vi "RefreshAutoUI.vi"(0 "TestDataRefs":refnum<vi>[](array[refnum]), 1 "RefreshAutoUIFunc":T3, 5 "CtrlPanelRefs":refnum<vi>[](array[refnum]), 7 "PIDCtrlRefs":refnum<vi>[](array[refnum]), 9 "OtherCtrlRefs":refnum<vi>[](array[refnum]), 11 "RecipeCtrlRefs":refnum<vi>[](array[refnum]), 12 "Setting":T1={"TorqueSensor"={"Interface"="", "Read Unit"=enum."Kg.cm", "Encoder"=0, "Torque Filter"=0, "Max Torque"=2.0, "Max Power"=50.0, "Max Speed"=50.0, "Scale Factor CW"=2.0, "Scale Factor CCW"=2.0, "Scale Factor Zero"=2.0}, "TorqueSensorL"={"Interface"="", "Read Unit"=enum."Kg.cm", "Encoder"=0, "Torque Filter"=0, "Max Torque"=2.0, "Max Power"=50.0, "Max Speed"=50.0, "Scale Factor CW"=2.0, "Scale Factor CCW"=2.0, "Scale Factor Zero"=2.0}, "Power Meter"={"Wiring"=0, "Interface"="", "1P Mode"=1, "1P CurrentLimit"=0.0, "3P Mode"=1, "3P CurrentLimit"=0.0}, "Thermocouple"={"Interface"="", "value range"="T/C T type -100 ~ 400 degree C", "Channel Count"=8, "Limit 0"=0.0, "Limit 1"=0.0, "Limit 2"=0.0, "Limit 3"=0.0, "Limit 4"=0.0, "Limit 5"=0.0, "Limit 6"=0.0, "Limit 7"=0.0}, "DC-1000"={"Interface"=enum."AD-1"}, "ServoMotor"={"Interface"=enum."AD-1"}, "MotorDriver"={"D_Interface"="", "L_Interface"=""}, "TestMode"=enum."電子中軸測試", "PowerSupply"={"Interface"="", "Current"=50.0, "Voltage"=50.0}} {"Thermocouple"."Limit 7" format="%.1f"; "Thermocouple"."Limit 6" format="%.1f"; "Thermocouple"."Limit 5" format="%.1f"; "Thermocouple"."Limit 4" format="%.1f"; "Thermocouple"."Limit 3" format="%.1f"; "Thermocouple"."Limit 2" format="%.1f"; "Thermocouple"."Limit 1" format="%.1f"; "Thermocouple"."Limit 0" format="%.1f"; "Thermocouple"."Channel Count" min=0 max=24; "Power Meter"."3P Mode" items=["RMS", "MEAN", "DC"]; "Power Meter"."1P Mode" items=["RMS", "MEAN", "DC"]; "Power Meter"."Wiring" items=["AD-0", "AD-1"]; "TorqueSensorL"."Scale Factor Zero" format="%#.6f"; "TorqueSensorL"."Scale Factor CCW" format="%#.6f"; "TorqueSensorL"."Scale Factor CW" format="%#.6f"; "TorqueSensorL"."Torque Filter" items=["OFF", "10Hz", "25Hz", "50Hz", "3Hz", "2Hz", "1Hz"]; "TorqueSensorL"."Encoder" items=["60-ppr"=60, "600-ppr"=600, "6000-ppr"=6000, "8192-ppr"=8192, "20-ppr"=20, "30-ppr"=30, "1-ppr"=1, "2-ppr"=2, "6-ppr"=6]; "TorqueSensor"."Scale Factor Zero" format="%#.6f"; "TorqueSensor"."Scale Factor CCW" format="%#.6f"; "TorqueSensor"."Scale Factor CW" format="%#.6f"; "TorqueSensor"."Torque Filter" items=["OFF", "10Hz", "25Hz", "50Hz", "3Hz", "2Hz", "1Hz"]; "TorqueSensor"."Encoder" items=["60-ppr"=60, "600-ppr"=600, "6000-ppr"=6000, "8192-ppr"=8192, "20-ppr"=20, "30-ppr"=30, "1-ppr"=1, "2-ppr"=2, "6-ppr"=6]}) -> ()   [LabVIEW 2024]
uses:
  RefreshAutoUIFunc.ctl
  MFActor/SystemSettings.ctl
panel:
  in  "Tab Control":T2(tab)
  in  "TestDataCurve":refnum<vi>
  in  "YAxis":refnum<vi>
  in  "XAxis":refnum<vi>
  in  "tbTestData":refnum<vi>
  in  "PIDGraph":refnum<vi>
  in  "pgTestData":refnum<vi>
  in  "ZeroLoadTorque":refnum<vi>
  in  "ZeroDriveTorque":refnum<vi>
  in  "ZeroDriveSpeed":refnum<vi>
  in  "LoadServoOn":refnum<vi>
  in  "DriveServoOn":refnum<vi>
  in  "TQOutput_L":refnum<vi>
  in  "SpeedOutput_D":refnum<vi>
  in  "CWCCW":refnum<vi>
  in  "pgCtrlPanel":refnum<vi>
  in  "TQOutput_D":refnum<vi>
  in  "OkeyForPID":refnum<vi>
  in  "PID Adj.End":refnum<vi>
  in  "PID Adj.Start":refnum<vi>
  in  "Close Loop Value Lo":refnum<vi>
  in  "Close Loop Value Hi":refnum<vi>
  in  "Close Loop Value Dwell":refnum<vi>
  in  "Close Loop Value Speed":refnum<vi>
  in  "NDS":refnum<vi>
  in  "NIS":refnum<vi>
  in  "NPS":refnum<vi>
  in  "ND":refnum<vi>
  in  "NI":refnum<vi>
  in  "NP":refnum<vi>
  in  "StopTest":refnum<vi>
  in  "StartTest":refnum<vi>
  in  "GotoCurvePage":refnum<vi>
  in  "GotoDataPage":refnum<vi>
  in  "ZeroDegree":refnum<vi>
  in  "ProcessConfirm":refnum<vi>
  in  "DynoValue_Auto":refnum<vi>
  in  "TestPanel":refnum<vi>
  in  "Trugh":refnum<vi>
  in  "LoadSideTQ":refnum<vi>
  in  "SinWaveTestSpeed":refnum<vi>
  in  "DegSetValue":refnum<vi>
  in  "TorqueSettingValue":refnum<vi>
  in  "Crest":refnum<vi>
  in  "PIDAdj":refnum<vi>
  in  "PID":refnum<vi>
  in  "MultiPtInitSpeed":refnum<vi>
  in  "Remove Button":refnum<vi>
  in  "Insert Button":refnum<vi>
  in  "Modify Button":refnum<vi>
  in  "Add Button":refnum<vi>
  in  "mtpTorque":refnum<vi>
  in  "mtpFetchRate":refnum<vi>
  in  "mtpDwellTime":refnum<vi>
  in  "mtpSpeed":refnum<vi>
  in  "idx":refnum<vi>
  in  "Program_Multi":refnum<vi>
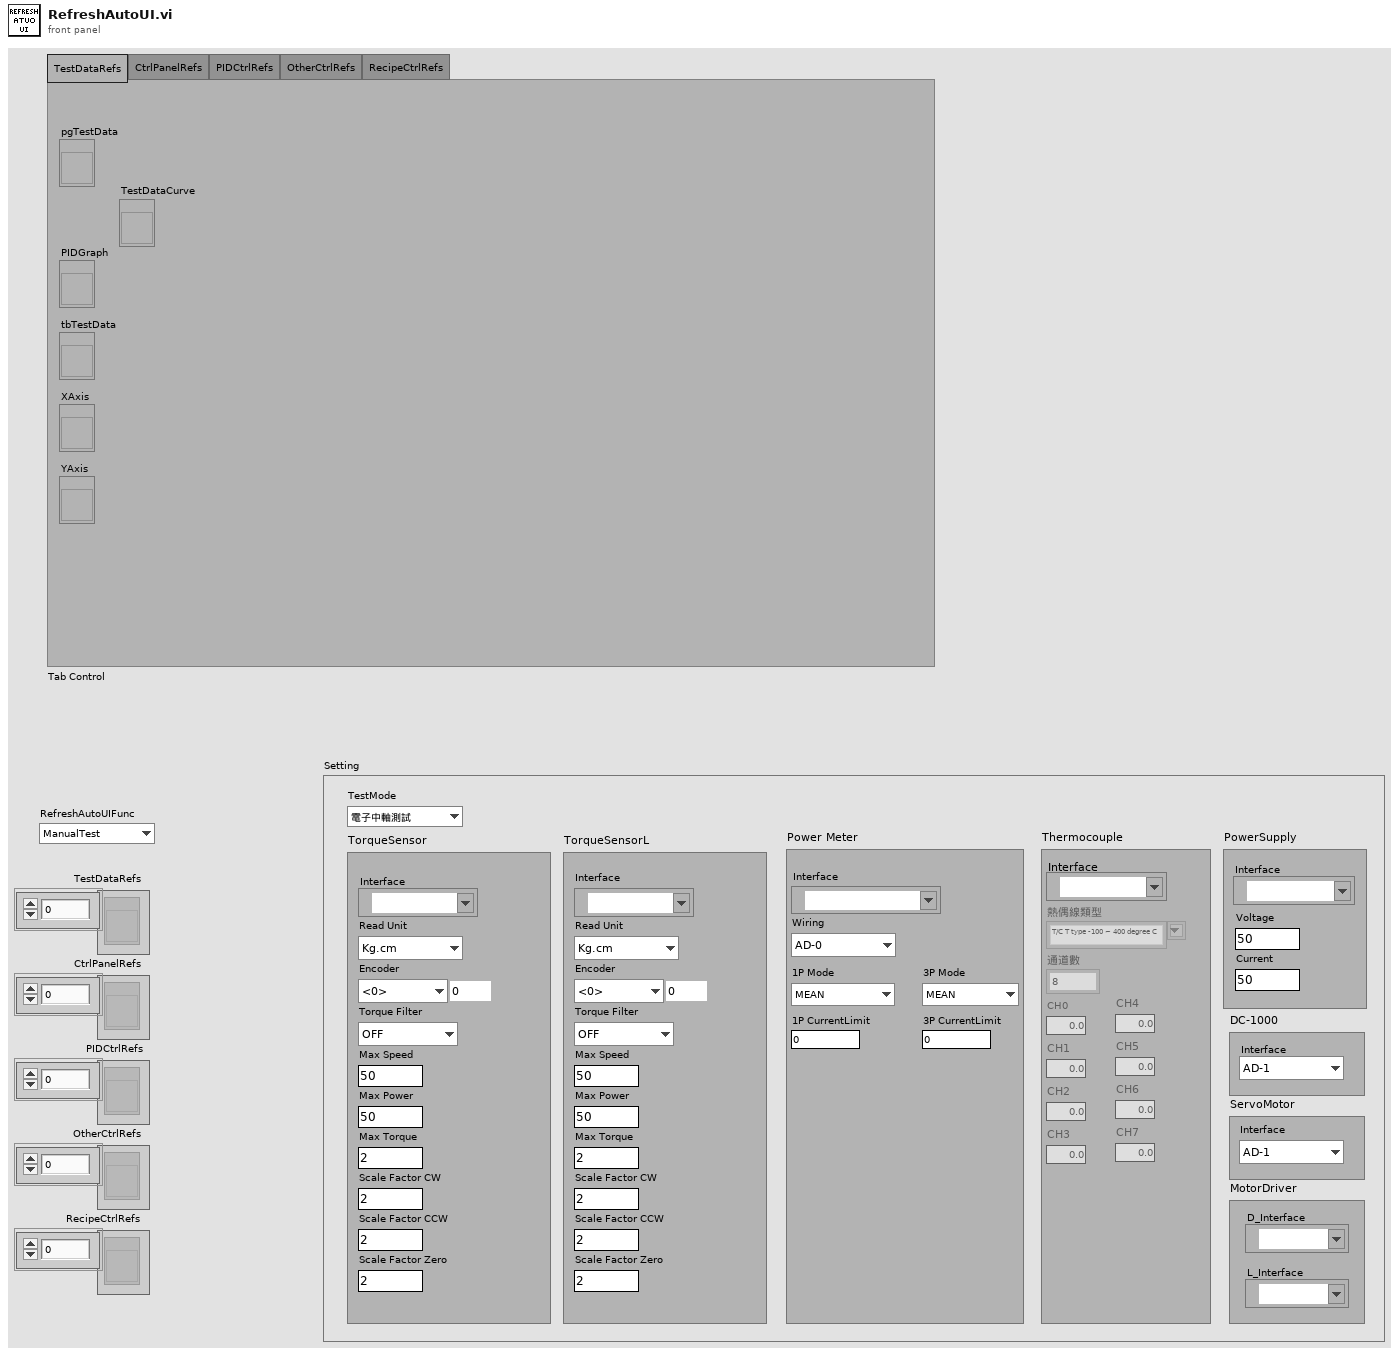
[diagram p1: front panel]
types:
  T1 = typedef "SystemSettings.ctl" = cluster{"TorqueSensor":cluster{"Interface":refnum<visa-resource-name>, "Read Unit":enum16{"oz.in", "oz.ft", "lb.in", "lb.ft", "g.cm", "Kg.cm", "mN.m", "cN.m", "N.m"}, "Encoder":u16, "Torque Filter":u16, "Max Torque":dbl, "Max Power":dbl, "Max Speed":dbl, "Scale Factor CW":dbl, "Scale Factor CCW":dbl, "Scale Factor Zero":dbl}, "TorqueSensorL":cluster{"Interface":refnum<visa-resource-name>, "Read Unit":enum16{"oz.in", "oz.ft", "lb.in", "lb.ft", "g.cm", "Kg.cm", "mN.m", "cN.m", "N.m"}, "Encoder":u16, "Torque Filter":u16, "Max Torque":dbl, "Max Power":dbl, "Max Speed":dbl, "Scale Factor CW":dbl, "Scale Factor CCW":dbl, "Scale Factor Zero":dbl}, "Power Meter":cluster{"Wiring":u16, "Interface":refnum<visa-resource-name>, "1P Mode":u16, "1P CurrentLimit":dbl, "3P Mode":u16, "3P CurrentLimit":dbl}, "Thermocouple":cluster{"Interface":refnum<visa-resource-name>, "value range":string, "Channel Count":i32, "Limit 0":dbl, "Limit 1":dbl, "Limit 2":dbl, "Limit 3":dbl, "Limit 4":dbl, "Limit 5":dbl, "Limit 6":dbl, "Limit 7":dbl}, "DC-1000":cluster{"Interface":enum16{"AD-0", "AD-1"}}, "ServoMotor":cluster{"Interface":enum16{"AD-0", "AD-1"}}, "MotorDriver":cluster{"D_Interface":refnum<visa-resource-name>, "L_Interface":refnum<visa-resource-name>}, "TestMode":enum16{"電子中軸測試", "中置電機測試"}, "PowerSupply":cluster{"Interface":refnum<visa-resource-name>, "Current":dbl, "Voltage":dbl}}
  T2 = enum32{"TestDataRefs", "CtrlPanelRefs", "PIDCtrlRefs", "OtherCtrlRefs", "RecipeCtrlRefs"}
  T3 = typedef "RefreshAutoUIFunc.ctl" = enum16{"ManualTest", "AngleMode", "LoadWaveCtrlMode", "DriveWaveCtrlMode", "EditMultiPt", "MultiPtTestMode", "FixPtTestMode", "AdjPID", "ConfirmBtnPos"}
  T4 = enum8{"Enabled", "Disabled", "Disabled and Grayed Out"}
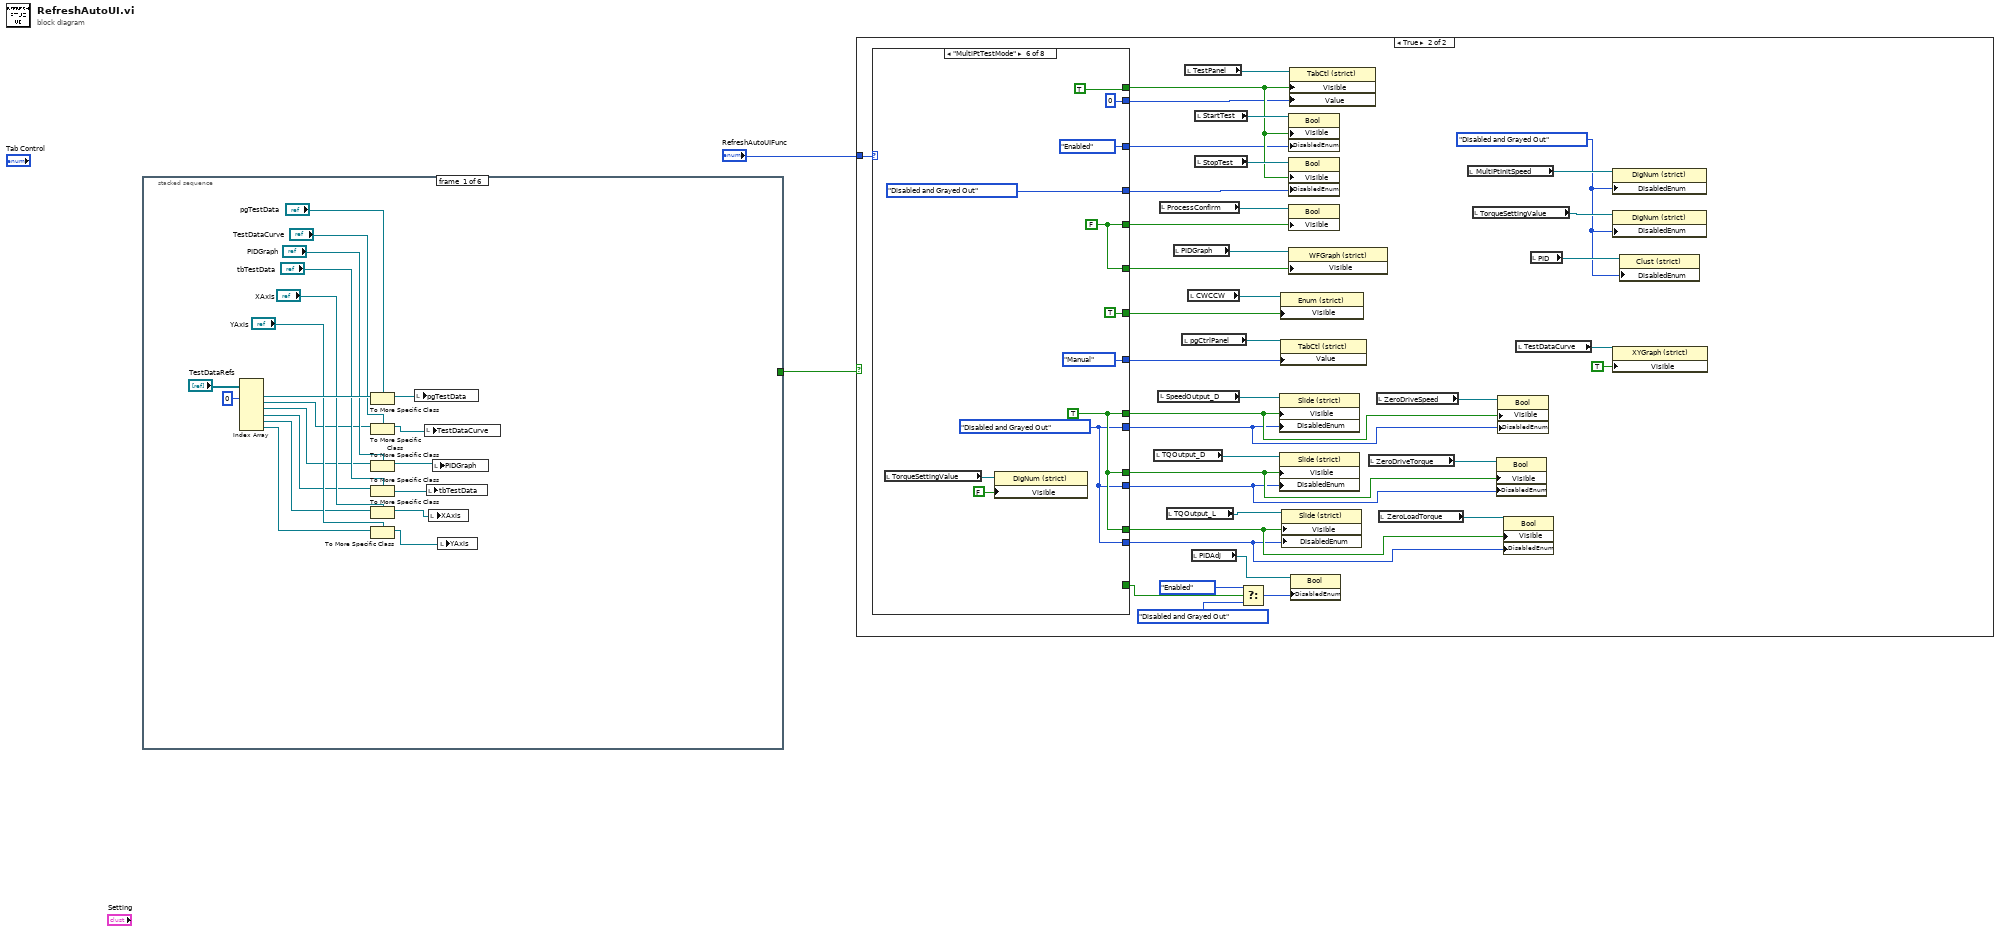
[diagram p0: block diagram]
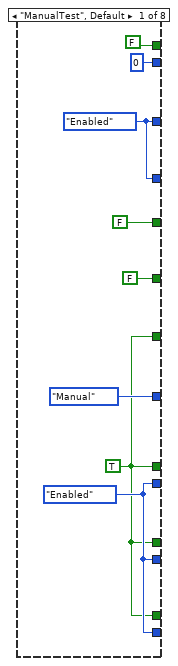
[diagram p3: hidden frame]
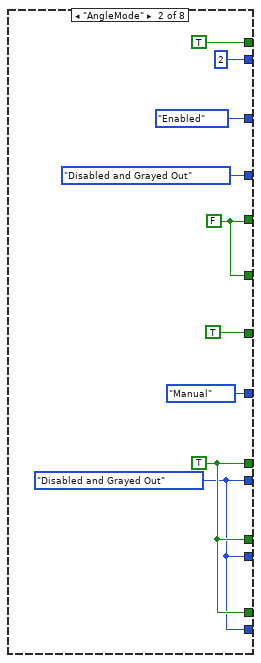
[diagram p4: hidden frame]
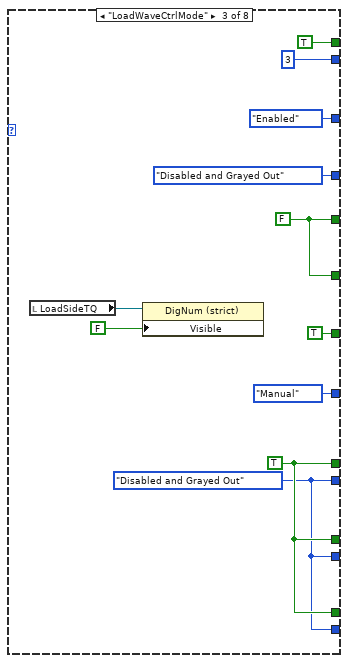
[diagram p5: hidden frame]
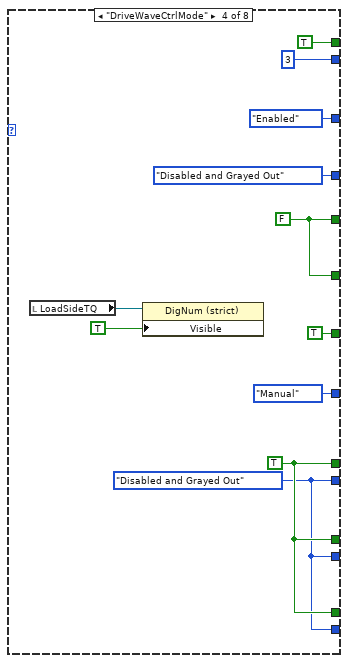
[diagram p6: hidden frame]
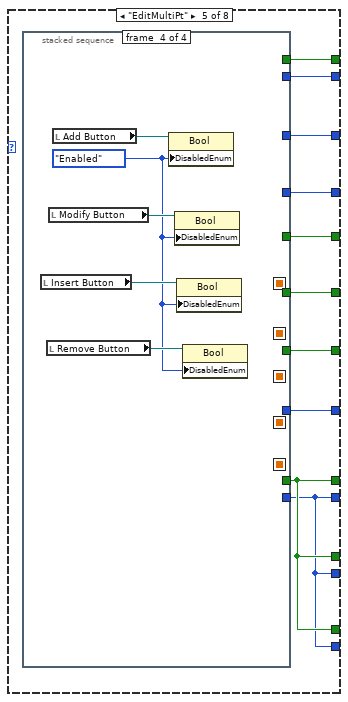
[diagram p7: hidden frame]
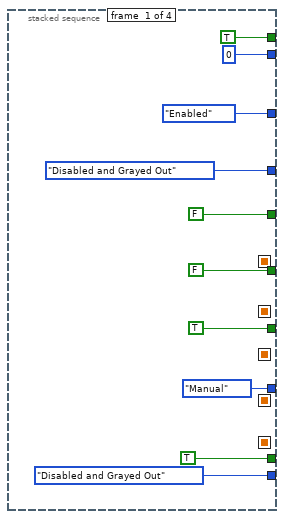
[diagram p8: hidden frame]
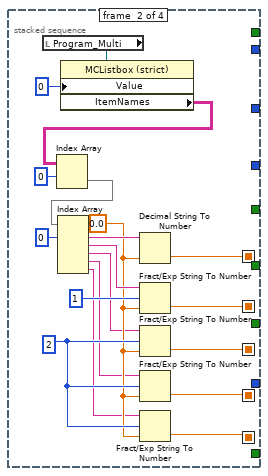
[diagram p9: hidden frame]
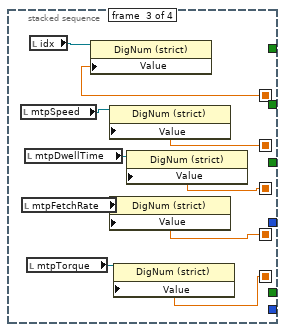
[diagram p10: hidden frame]
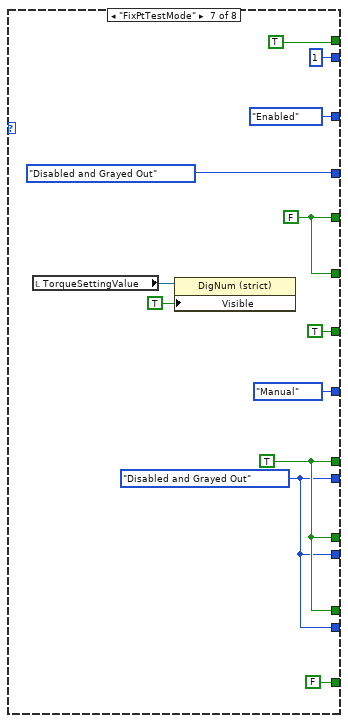
[diagram p11: hidden frame]
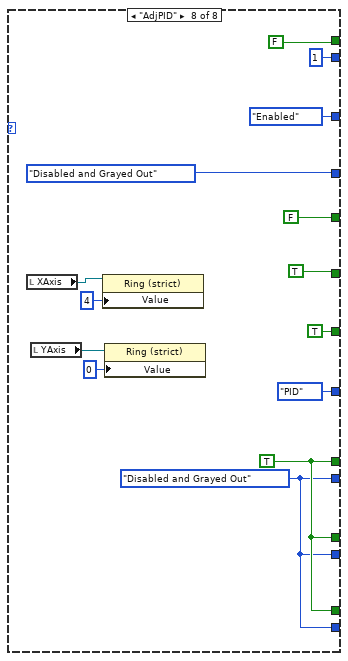
[diagram p12: hidden frame]
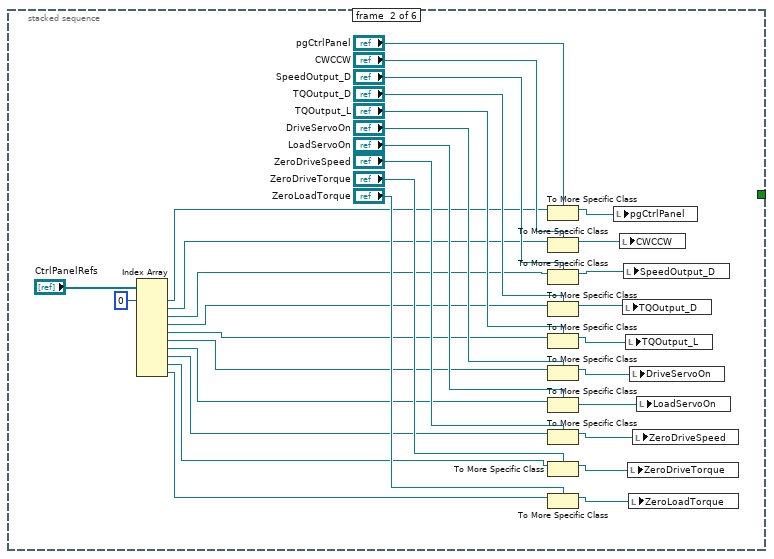
[diagram p13: hidden frame]
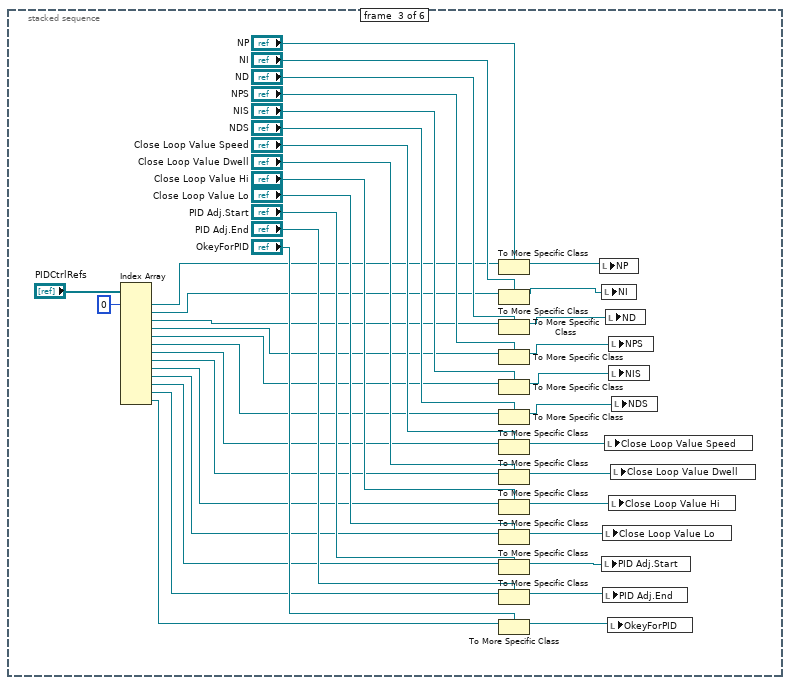
[diagram p14: hidden frame]
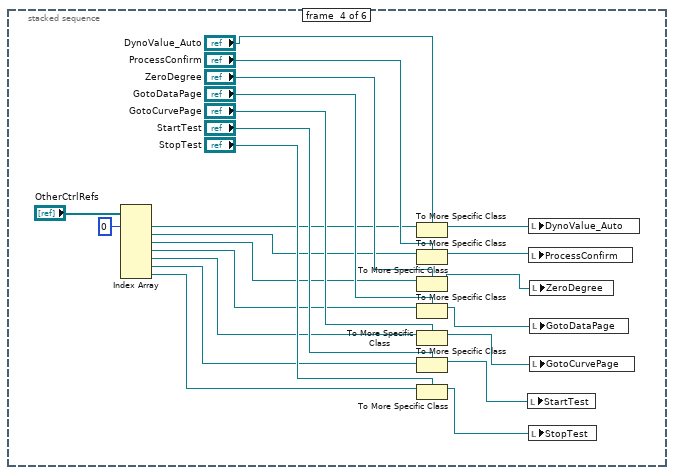
[diagram p15: hidden frame]
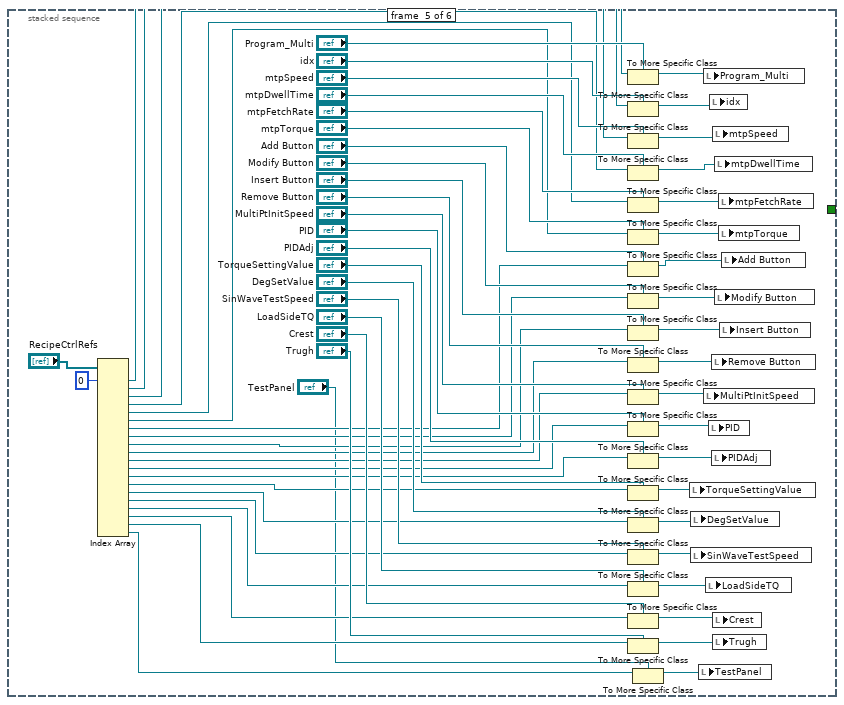
[diagram p16: hidden frame]
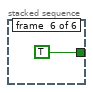
[diagram p17: hidden frame]
diagram:
  n1 = stacked-sequence {
    tunnel: [_ _ _ _ _ TRUE] -> w2
    frame #0 {
      n2 = Index Array(array="TestDataRefs", index #1=0 ("index")) -> (element #1=w20:refnum<vi>, element #2=w3:refnum<vi>, element #3=w4:refnum<vi>, element #4=w5:refnum<vi>, element #5=w6:refnum<vi>, element #6=w7:refnum<vi>)  [unwired: 5 in]
      n3 = To More Specific Class(target class="pgTestData", reference=w20) -> (specific class reference=w19:refnum<vi>)  [unwired: 1 in, 1 out]
      n4 = To More Specific Class(target class="TestDataCurve", reference=w3) -> (specific class reference=w9:refnum<vi>)  [unwired: 1 in, 1 out]
      n5 = To More Specific Class(target class="PIDGraph", reference=w4) -> (specific class reference=w15:refnum<vi>)  [unwired: 1 in, 1 out]
      n6 = To More Specific Class(target class="tbTestData", reference=w5) -> (specific class reference=w14:refnum<vi>)  [unwired: 1 in, 1 out]
      n7 = To More Specific Class(target class="XAxis", reference=w6) -> (specific class reference=w13:refnum<vi>)  [unwired: 1 in, 1 out]
      n8 = To More Specific Class(target class="YAxis", reference=w7) -> (specific class reference=w12:refnum<vi>)  [unwired: 1 in, 1 out]
      n9 = local write "pgTestData"(w19) -> ()
      n10 = local write "TestDataCurve"(w9) -> ()
      n11 = local write "tbTestData"(w14) -> ()
      n12 = local write "XAxis"(w13) -> ()
      n13 = local write "PIDGraph"(w15) -> ()
      n14 = local write "YAxis"(w12) -> ()
    }
    frame #1 {
      n15 = Index Array(array="CtrlPanelRefs", index #1=0 ("index")) -> (element #1=w32:refnum<vi>, element #2=w31:refnum<vi>, element #3=w30:refnum<vi>, element #4=w29:refnum<vi>, element #5=w28:refnum<vi>, element #6=w27:refnum<vi>, element #7=w26:refnum<vi>, element #8=w25:refnum<vi>, element #9=w24:refnum<vi>, element #10=w23:refnum<vi>)  [unwired: 9 in]
      n16 = To More Specific Class(target class="pgCtrlPanel", reference=w32) -> (specific class reference=w42:refnum<vi>)  [unwired: 1 in, 1 out]
      n17 = To More Specific Class(target class="CWCCW", reference=w31) -> (specific class reference=w41:refnum<vi>)  [unwired: 1 in, 1 out]
      n18 = To More Specific Class(target class="SpeedOutput_D", reference=w30) -> (specific class reference=w40:refnum<vi>)  [unwired: 1 in, 1 out]
      n19 = To More Specific Class(target class="TQOutput_D", reference=w29) -> (specific class reference=w39:refnum<vi>)  [unwired: 1 in, 1 out]
      n20 = To More Specific Class(target class="TQOutput_L", reference=w28) -> (specific class reference=w38:refnum<vi>)  [unwired: 1 in, 1 out]
      n21 = To More Specific Class(target class="DriveServoOn", reference=w27) -> (specific class reference=w37:refnum<vi>)  [unwired: 1 in, 1 out]
      n22 = To More Specific Class(target class="LoadServoOn", reference=w26) -> (specific class reference=w36:refnum<vi>)  [unwired: 1 in, 1 out]
      n23 = To More Specific Class(target class="ZeroDriveSpeed", reference=w25) -> (specific class reference=w35:refnum<vi>)  [unwired: 1 in, 1 out]
      n24 = To More Specific Class(target class="ZeroDriveTorque", reference=w24) -> (specific class reference=w34:refnum<vi>)  [unwired: 1 in, 1 out]
      n25 = To More Specific Class(target class="ZeroLoadTorque", reference=w23) -> (specific class reference=w33:refnum<vi>)  [unwired: 1 in, 1 out]
      n26 = local write "pgCtrlPanel"(w42) -> ()
      n27 = local write "CWCCW"(w41) -> ()
      n28 = local write "TQOutput_D"(w39) -> ()
      n29 = local write "SpeedOutput_D"(w40) -> ()
      n30 = local write "TQOutput_L"(w38) -> ()
      n31 = local write "ZeroDriveTorque"(w34) -> ()
      n32 = local write "ZeroLoadTorque"(w33) -> ()
      n33 = local write "DriveServoOn"(w37) -> ()
      n34 = local write "ZeroDriveSpeed"(w35) -> ()
      n35 = local write "LoadServoOn"(w36) -> ()
    }
    frame #2 {
      n36 = Index Array(array="PIDCtrlRefs", index #1=0 ("index")) -> (element #1=w80:refnum<vi>, element #2=w79:refnum<vi>, element #3=w78:refnum<vi>, element #4=w77:refnum<vi>, element #5=w76:refnum<vi>, element #6=w75:refnum<vi>, element #7=w74:refnum<vi>, element #8=w73:refnum<vi>, element #9=w72:refnum<vi>, element #10=w71:refnum<vi>, element #11=w70:refnum<vi>, element #12=w69:refnum<vi>, element #13=w68:refnum<vi>)  [unwired: 12 in]
      n37 = To More Specific Class(target class="NP", reference=w80) -> (specific class reference=w67:refnum<vi>)  [unwired: 1 in, 1 out]
      n38 = To More Specific Class(target class="NI", reference=w79) -> (specific class reference=w66:refnum<vi>)  [unwired: 1 in, 1 out]
      n39 = To More Specific Class(target class="ND", reference=w78) -> (specific class reference=w65:refnum<vi>)  [unwired: 1 in, 1 out]
      n40 = To More Specific Class(target class="NPS", reference=w77) -> (specific class reference=w64:refnum<vi>)  [unwired: 1 in, 1 out]
      n41 = To More Specific Class(target class="NIS", reference=w76) -> (specific class reference=w63:refnum<vi>)  [unwired: 1 in, 1 out]
      n42 = To More Specific Class(target class="NDS", reference=w75) -> (specific class reference=w62:refnum<vi>)  [unwired: 1 in, 1 out]
      n43 = To More Specific Class(target class="Close Loop Value Speed", reference=w74) -> (specific class reference=w61:refnum<vi>)  [unwired: 1 in, 1 out]
      n44 = To More Specific Class(target class="Close Loop Value Dwell", reference=w73) -> (specific class reference=w60:refnum<vi>)  [unwired: 1 in, 1 out]
      n45 = To More Specific Class(target class="Close Loop Value Hi", reference=w72) -> (specific class reference=w59:refnum<vi>)  [unwired: 1 in, 1 out]
      n46 = To More Specific Class(target class="Close Loop Value Lo", reference=w71) -> (specific class reference=w58:refnum<vi>)  [unwired: 1 in, 1 out]
      n47 = To More Specific Class(target class="PID Adj.Start", reference=w70) -> (specific class reference=w57:refnum<vi>)  [unwired: 1 in, 1 out]
      n48 = To More Specific Class(target class="PID Adj.End", reference=w69) -> (specific class reference=w56:refnum<vi>)  [unwired: 1 in, 1 out]
      n49 = To More Specific Class(target class="OkeyForPID", reference=w68) -> (specific class reference=w55:refnum<vi>)  [unwired: 1 in, 1 out]
      n50 = local write "NP"(w67) -> ()
      n51 = local write "NI"(w66) -> ()
      n52 = local write "PID Adj.Start"(w57) -> ()
      n53 = local write "Close Loop Value Lo"(w58) -> ()
      n54 = local write "PID Adj.End"(w56) -> ()
      n55 = local write "Close Loop Value Speed"(w61) -> ()
      n56 = local write "ND"(w65) -> ()
      n57 = local write "OkeyForPID"(w55) -> ()
      n58 = local write "NPS"(w64) -> ()
      n59 = local write "NIS"(w63) -> ()
      n60 = local write "Close Loop Value Hi"(w59) -> ()
      n61 = local write "Close Loop Value Dwell"(w60) -> ()
      n62 = local write "NDS"(w62) -> ()
    }
    frame #3 {
      n63 = Index Array(array="OtherCtrlRefs", index #1=0 ("index")) -> (element #1=w109:refnum<vi>, element #2=w108:refnum<vi>, element #3=w107:refnum<vi>, element #4=w106:refnum<vi>, element #5=w105:refnum<vi>, element #6=w104:refnum<vi>, element #7=w103:refnum<vi>)  [unwired: 6 in]
      n64 = To More Specific Class(target class="DynoValue_Auto", reference=w109) -> (specific class reference=w102:refnum<vi>)  [unwired: 1 in, 1 out]
      n65 = To More Specific Class(target class="ProcessConfirm", reference=w108) -> (specific class reference=w101:refnum<vi>)  [unwired: 1 in, 1 out]
      n66 = To More Specific Class(target class="ZeroDegree", reference=w107) -> (specific class reference=w100:refnum<vi>)  [unwired: 1 in, 1 out]
      n67 = To More Specific Class(target class="GotoDataPage", reference=w106) -> (specific class reference=w99:refnum<vi>)  [unwired: 1 in, 1 out]
      n68 = To More Specific Class(target class="GotoCurvePage", reference=w105) -> (specific class reference=w98:refnum<vi>)  [unwired: 1 in, 1 out]
      n69 = To More Specific Class(target class="StartTest", reference=w104) -> (specific class reference=w97:refnum<vi>)  [unwired: 1 in, 1 out]
      n70 = To More Specific Class(target class="StopTest", reference=w103) -> (specific class reference=w96:refnum<vi>)  [unwired: 1 in, 1 out]
      n71 = local write "StartTest"(w97) -> ()
      n72 = local write "DynoValue_Auto"(w102) -> ()
      n73 = local write "ProcessConfirm"(w101) -> ()
      n74 = local write "StopTest"(w96) -> ()
      n75 = local write "ZeroDegree"(w100) -> ()
      n76 = local write "GotoDataPage"(w99) -> ()
      n77 = local write "GotoCurvePage"(w98) -> ()
    }
    frame #4 {
      n78 = Index Array(array="RecipeCtrlRefs", index #1=0 ("index")) -> (element #1=w159:refnum<vi>, element #2=w158:refnum<vi>, element #3=w157:refnum<vi>, element #4=w156:refnum<vi>, element #5=w155:refnum<vi>, element #6=w154:refnum<vi>, element #7=w153:refnum<vi>, element #8=w152:refnum<vi>, element #9=w151:refnum<vi>, element #10=w150:refnum<vi>, element #11=w149:refnum<vi>, element #12=w148:refnum<vi>, element #13=w147:refnum<vi>, element #14=w146:refnum<vi>, element #15=w145:refnum<vi>, element #16=w144:refnum<vi>, element #17=w143:refnum<vi>, element #18=w142:refnum<vi>, element #19=w141:refnum<vi>, element #20=w120:refnum<vi>)  [unwired: 19 in]
      n79 = To More Specific Class(target class="Program_Multi", reference=w159) -> (specific class reference=w140:refnum<vi>)  [unwired: 1 in, 1 out]
      n80 = To More Specific Class(target class="idx", reference=w158) -> (specific class reference=w139:refnum<vi>)  [unwired: 1 in, 1 out]
      n81 = To More Specific Class(target class="mtpSpeed", reference=w157) -> (specific class reference=w138:refnum<vi>)  [unwired: 1 in, 1 out]
      n82 = To More Specific Class(target class="mtpDwellTime", reference=w156) -> (specific class reference=w137:refnum<vi>)  [unwired: 1 in, 1 out]
      n83 = To More Specific Class(target class="mtpFetchRate", reference=w155) -> (specific class reference=w136:refnum<vi>)  [unwired: 1 in, 1 out]
      n84 = To More Specific Class(target class="mtpTorque", reference=w154) -> (specific class reference=w135:refnum<vi>)  [unwired: 1 in, 1 out]
      n85 = To More Specific Class(target class="Add Button", reference=w153) -> (specific class reference=w134:refnum<vi>)  [unwired: 1 in, 1 out]
      n86 = To More Specific Class(target class="Modify Button", reference=w152) -> (specific class reference=w133:refnum<vi>)  [unwired: 1 in, 1 out]
      n87 = To More Specific Class(target class="Insert Button", reference=w151) -> (specific class reference=w132:refnum<vi>)  [unwired: 1 in, 1 out]
      n88 = To More Specific Class(target class="Remove Button", reference=w150) -> (specific class reference=w131:refnum<vi>)  [unwired: 1 in, 1 out]
      n89 = To More Specific Class(target class="MultiPtInitSpeed", reference=w149) -> (specific class reference=w130:refnum<vi>)  [unwired: 1 in, 1 out]
      n90 = To More Specific Class(target class="PID", reference=w148) -> (specific class reference=w129:refnum<vi>)  [unwired: 1 in, 1 out]
      n91 = To More Specific Class(target class="PIDAdj", reference=w147) -> (specific class reference=w128:refnum<vi>)  [unwired: 1 in, 1 out]
      n92 = To More Specific Class(target class="TorqueSettingValue", reference=w146) -> (specific class reference=w127:refnum<vi>)  [unwired: 1 in, 1 out]
      n93 = To More Specific Class(target class="DegSetValue", reference=w145) -> (specific class reference=w126:refnum<vi>)  [unwired: 1 in, 1 out]
      n94 = To More Specific Class(target class="SinWaveTestSpeed", reference=w144) -> (specific class reference=w125:refnum<vi>)  [unwired: 1 in, 1 out]
      n95 = To More Specific Class(target class="LoadSideTQ", reference=w143) -> (specific class reference=w124:refnum<vi>)  [unwired: 1 in, 1 out]
      n96 = To More Specific Class(target class="Crest", reference=w142) -> (specific class reference=w123:refnum<vi>)  [unwired: 1 in, 1 out]
      n97 = To More Specific Class(target class="Trugh", reference=w141) -> (specific class reference=w122:refnum<vi>)  [unwired: 1 in, 1 out]
      n98 = To More Specific Class(target class="TestPanel", reference=w120) -> (specific class reference=w119:refnum<vi>)  [unwired: 1 in, 1 out]
      n99 = local write "TorqueSettingValue"(w127) -> ()
      n100 = local write "DegSetValue"(w126) -> ()
      n101 = local write "SinWaveTestSpeed"(w125) -> ()
      n102 = local write "TestPanel"(w119) -> ()
      n103 = local write "Program_Multi"(w140) -> ()
      n104 = local write "MultiPtInitSpeed"(w130) -> ()
      n105 = local write "LoadSideTQ"(w124) -> ()
      n106 = local write "PID"(w129) -> ()
      n107 = local write "idx"(w139) -> ()
      n108 = local write "Remove Button"(w131) -> ()
      n109 = local write "PIDAdj"(w128) -> ()
      n110 = local write "mtpSpeed"(w138) -> ()
      n111 = local write "Crest"(w123) -> ()
      n112 = local write "Trugh"(w122) -> ()
      n113 = local write "mtpDwellTime"(w137) -> ()
      n114 = local write "Modify Button"(w133) -> ()
      n115 = local write "mtpFetchRate"(w136) -> ()
      n116 = local write "mtpTorque"(w135) -> ()
      n117 = local write "Insert Button"(w132) -> ()
      n118 = local write "Add Button"(w134) -> ()
    }
    frame #5 {
    }
  }
  n119 = case shown="True" w2 {
    tunnel: "RefreshAutoUIFunc" -> [_ w220]
    frame False {
    }
    frame True {
      w184 = T4."Disabled and Grayed Out" ("Disabled")
      n120 = case shown="\"MultiPtTestMode\"" w220 {
        tunnel: [FALSE TRUE TRUE TRUE w269 TRUE TRUE FALSE] -> w215
        tunnel: [FALSE w233 w244 w255 w265 w321 w333 TRUE] -> w213
        tunnel: [enum32{"Manual", "PID"}."Manual" ("Value") enum32{"Manual", "PID"}."Manual" ("Value") enum32{"Manual", "PID"}."Manual" ("Value") enum32{"Manual", "PID"}."Manual" ("Value") w263 enum32{"Manual", "PID"}."Manual" ("Value") enum32{"Manual", "PID"}."Manual" ("Value") enum32{"Manual", "PID"}."PID" ("Value")] -> w211
        tunnel: [w224 w231 w241 w252 w262 w318 w330 w344] -> w204
        tunnel: [w224 w231 w241 w252 w262 w318 w330 w344] -> w202
        tunnel: [w224 w231 w241 w252 w262 w318 w330 w344] -> w200
        tunnel: [w225 w230 w240 w251 w261 w317 w329 w343] -> w203
        tunnel: [w225 w230 w240 w251 w261 w317 w329 w343] -> w201
        tunnel: [w225 w230 w240 w251 w261 w317 w329 w343] -> w199
        tunnel: [w224 TRUE TRUE TRUE w264 TRUE TRUE TRUE] -> w197
        tunnel: [FALSE w233 w244 w255 w266 w321 w333 FALSE] -> w196
        tunnel: [u32 0 u32 2 u32 3 u32 3 w268 u32 0 u32 1 u32 1] -> w195
        tunnel: [w221 T4."Enabled" ("Disabled") T4."Enabled" ("Disabled") T4."Enabled" ("Disabled") w267 T4."Enabled" ("Disabled") T4."Enabled" ("Disabled") T4."Enabled" ("Disabled")] -> w194
        tunnel: [w221 T4."Disabled and Grayed Out" ("Disabled") T4."Disabled and Grayed Out" ("Disabled") T4."Disabled and Grayed Out" ("Disabled") w260 T4."Disabled and Grayed Out" ("Disabled") T4."Disabled and Grayed Out" ("Disabled") T4."Disabled and Grayed Out" ("Disabled")] -> w193
        tunnel: [_ _ _ _ _ _ FALSE _] -> w190
        frame "ManualTest", Default {
          w221 = T4."Enabled" ("Disabled")
          w225 = T4."Enabled" ("Disabled")
          w224 = TRUE
        }
        frame "AngleMode" {
          w230 = T4."Disabled and Grayed Out" ("Disabled")
          w231 = TRUE
          w233 = FALSE
        }
        frame "LoadWaveCtrlMode" {
          w240 = T4."Disabled and Grayed Out" ("Disabled")
          w241 = TRUE
          w244 = FALSE
          n121 = local read "LoadSideTQ"() -> (w239:refnum<vi>)
          n122 = property class="DigNum (strict)"(reference=w239, "Visible"=FALSE) -> ()  [unwired: 1 in, 2 out]
        }
        frame "DriveWaveCtrlMode" {
          w251 = T4."Disabled and Grayed Out" ("Disabled")
          w252 = TRUE
          w255 = FALSE
          n123 = local read "LoadSideTQ"() -> (w250:refnum<vi>)
          n124 = property class="DigNum (strict)"(reference=w250, "Visible"=TRUE) -> ()  [unwired: 1 in, 2 out]
        }
        frame "EditMultiPt" {
          n125 = stacked-sequence {
            seq-local: [_ w287 _ _] -> [_ _ w307 _]
            seq-local: [_ w286 _ _] -> [_ _ w305 _]
            seq-local: [_ w285 _ _] -> [_ _ w303 _]
            seq-local: [_ w284 _ _] -> [_ _ w301 _]
            seq-local: [_ w283 _ _] -> [_ _ w299 _]
            tunnel: [TRUE _ _ _] -> w269
            tunnel: [u32 0 _ _ _] -> w268
            tunnel: [T4."Enabled" ("Disabled") _ _ _] -> w267
            tunnel: [FALSE _ _ _] -> w266
            tunnel: [FALSE _ _ _] -> w265
            tunnel: [TRUE _ _ _] -> w264
            tunnel: [enum32{"Manual", "PID"}."Manual" ("Value") _ _ _] -> w263
            tunnel: [TRUE _ _ _] -> w262
            tunnel: [T4."Disabled and Grayed Out" ("Disabled") _ _ _] -> w261
            tunnel: [T4."Disabled and Grayed Out" ("Disabled") _ _ _] -> w260
            frame #0 {
            }
            frame #1 {
              w290 = 2 ("offset")
              w288 = 0.0 ("default (0 I32)")
              n126 = local read "Program_Multi"() -> (w298:refnum<vi>)
              n127 = property class="MCListbox (strict)"(reference=w298, "Value"=0) -> ("ItemNames"=w296:string[][])  [unwired: 1 in, 2 out]
              n128 = Index Array(array=w296, index (row)=0) -> (element=w294:string[])  [unwired: 1 in]
              n129 = Index Array(array=w294, index #1=0 ("index")) -> (element #1=w292:string, element #2=w289:string, element #3=w282:string, element #4=w281:string, element #5=w280:string)  [unwired: 4 in]
              n130 = Decimal String To Number(string=w292, default (0L)=w288) -> (number=w287:dbl)  [unwired: 1 in, 1 out]
              n131 = Fract/Exp String To Number(string=w289, offset=1, default (0 dbl)=w288) -> (number=w286:dbl)  [unwired: 1 in, 1 out]
              n132 = Fract/Exp String To Number(string=w282, offset=w290, default (0 dbl)=w288) -> (number=w285:dbl)  [unwired: 1 in, 1 out]
              n133 = Fract/Exp String To Number(string=w281, offset=w290, default (0 dbl)=w288) -> (number=w284:dbl)  [unwired: 1 in, 1 out]
              n134 = Fract/Exp String To Number(string=w280, offset=w290, default (0 dbl)=w288) -> (number=w283:dbl)  [unwired: 1 in, 1 out]
            }
            frame #2 {
              n135 = local read "mtpSpeed"() -> (w306:refnum<vi>)
              n136 = local read "mtpFetchRate"() -> (w302:refnum<vi>)
              n137 = local read "mtpDwellTime"() -> (w304:refnum<vi>)
              n138 = local read "mtpTorque"() -> (w300:refnum<vi>)
              n139 = local read "idx"() -> (w308:refnum<vi>)
              n140 = property class="DigNum (strict)"(reference=w308, "Value"=w307) -> ()  [unwired: 1 in, 2 out]
              n141 = property class="DigNum (strict)"(reference=w306, "Value"=w305) -> ()  [unwired: 1 in, 2 out]
              n142 = property class="DigNum (strict)"(reference=w302, "Value"=w301) -> ()  [unwired: 1 in, 2 out]
              n143 = property class="DigNum (strict)"(reference=w300, "Value"=w299) -> ()  [unwired: 1 in, 2 out]
              n144 = property class="DigNum (strict)"(reference=w304, "Value"=w303) -> ()  [unwired: 1 in, 2 out]
            }
            frame #3 {
              w309 = T4."Enabled" ("Disabled")
              n145 = local read "Insert Button"() -> (w311:refnum<vi>)
              n146 = local read "Remove Button"() -> (w310:refnum<vi>)
              n147 = local read "Modify Button"() -> (w312:refnum<vi>)
              n148 = local read "Add Button"() -> (w313:refnum<vi>)
              n149 = property class="Bool"(reference=w313, "DisabledEnum"=w309) -> ()  [unwired: 1 in, 2 out]
              n150 = property class="Bool"(reference=w312, "DisabledEnum"=w309) -> ()  [unwired: 1 in, 2 out]
              n151 = property class="Bool"(reference=w311, "DisabledEnum"=w309) -> ()  [unwired: 1 in, 2 out]
              n152 = property class="Bool"(reference=w310, "DisabledEnum"=w309) -> ()  [unwired: 1 in, 2 out]
            }
          }
        }
        frame "MultiPtTestMode" {
          w317 = T4."Disabled and Grayed Out" ("Disabled")
          w318 = TRUE
          w321 = FALSE
          n153 = local read "TorqueSettingValue"() -> (w315:refnum<vi>)
          n154 = property class="DigNum (strict)"(reference=w315, "Visible"=FALSE) -> ()  [unwired: 1 in, 2 out]
        }
        frame "FixPtTestMode" {
          w329 = T4."Disabled and Grayed Out" ("Disabled")
          w330 = TRUE
          w333 = FALSE
          n155 = local read "TorqueSettingValue"() -> (w327:refnum<vi>)
          n156 = property class="DigNum (strict)"(reference=w327, "Visible"=TRUE) -> ()  [unwired: 1 in, 2 out]
        }
        frame "AdjPID" {
          w343 = T4."Disabled and Grayed Out" ("Disabled")
          w344 = TRUE
          n157 = local read "XAxis"() -> (w340:refnum<vi>)
          n158 = local read "YAxis"() -> (w339:refnum<vi>)
          n159 = property class="Ring (strict)"(reference=w340, "Value"=u16 4) -> ()  [unwired: 1 in, 2 out]
          n160 = property class="Ring (strict)"(reference=w339, "Value"=u16 0) -> ()  [unwired: 1 in, 2 out]
        }
      }
      n161 = local read "TQOutput_D"() -> (w209:refnum<vi>)
      n162 = local read "SpeedOutput_D"() -> (w210:refnum<vi>)
      n163 = local read "ProcessConfirm"() -> (w216:refnum<vi>)
      n164 = local read "TQOutput_L"() -> (w208:refnum<vi>)
      n165 = local read "PIDGraph"() -> (w214:refnum<vi>)
      n166 = local read "pgCtrlPanel"() -> (w212:refnum<vi>)
      n167 = local read "TestPanel"() -> (w219:refnum<vi>)
      n168 = local read "CWCCW"() -> (w198:refnum<vi>)
      n169 = local read "PIDAdj"() -> (w192:refnum<vi>)
      n170 = local read "StartTest"() -> (w218:refnum<vi>)
      n171 = local read "StopTest"() -> (w217:refnum<vi>)
      n172 = Select(t=T4."Enabled" ("Disabled"), s=w190, f=T4."Disabled and Grayed Out" ("Disabled")) -> (s? t:f=w189:T4)
      n173 = property class="Slide (strict)"(reference=w210, "Visible"=w204, "DisabledEnum"=w203) -> ()  [unwired: 1 in, 2 out]
      n174 = property class="Slide (strict)"(reference=w209, "Visible"=w202, "DisabledEnum"=w201) -> ()  [unwired: 1 in, 2 out]
      n175 = property class="Enum (strict)"(reference=w198, "Visible"=w197) -> ()  [unwired: 1 in, 2 out]
      n176 = property class="TabCtl (strict)"(reference=w212, "Value"=w211) -> ()  [unwired: 1 in, 2 out]
      n177 = property class="Slide (strict)"(reference=w208, "Visible"=w200, "DisabledEnum"=w199) -> ()  [unwired: 1 in, 2 out]
      n178 = property class="Bool"(reference=w218, "Visible"=w215, "DisabledEnum"=w194) -> ()  [unwired: 1 in, 2 out]
      n179 = property class="Bool"(reference=w217, "Visible"=w215, "DisabledEnum"=w193) -> ()  [unwired: 1 in, 2 out]
      n180 = property class="Bool"(reference=w216, "Visible"=w196) -> ()  [unwired: 1 in, 2 out]
      n181 = property class="WFGraph (strict)"(reference=w214, "Visible"=w213) -> ()  [unwired: 1 in, 2 out]
      n182 = property class="TabCtl (strict)"(reference=w219, "Visible"=w215, "Value"=w195) -> ()  [unwired: 1 in, 2 out]
      n183 = property class="Bool"(reference=w192, "DisabledEnum"=w189) -> ()  [unwired: 1 in, 2 out]
      n184 = local read "ZeroDriveTorque"() -> (w206:refnum<vi>)
      n185 = local read "ZeroDriveSpeed"() -> (w207:refnum<vi>)
      n186 = local read "ZeroLoadTorque"() -> (w205:refnum<vi>)
      n187 = local read "MultiPtInitSpeed"() -> (w187:refnum<vi>)
      n188 = local read "TorqueSettingValue"() -> (w186:refnum<vi>)
      n189 = property class="Bool"(reference=w206, "Visible"=w202, "DisabledEnum"=w201) -> ()  [unwired: 1 in, 2 out]
      n190 = property class="Bool"(reference=w207, "Visible"=w204, "DisabledEnum"=w203) -> ()  [unwired: 1 in, 2 out]
      n191 = property class="Bool"(reference=w205, "Visible"=w200, "DisabledEnum"=w199) -> ()  [unwired: 1 in, 2 out]
      n192 = local read "TestDataCurve"() -> (w183:refnum<vi>)
      n193 = local read "PID"() -> (w185:refnum<vi>)
      n194 = property class="DigNum (strict)"(reference=w187, "DisabledEnum"=w184) -> ()  [unwired: 1 in, 2 out]
      n195 = property class="DigNum (strict)"(reference=w186, "DisabledEnum"=w184) -> ()  [unwired: 1 in, 2 out]
      n196 = property class="XYGraph (strict)"(reference=w183, "Visible"=TRUE) -> ()  [unwired: 1 in, 2 out]
      n197 = property class="Clust (strict)"(reference=w185, "DisabledEnum"=w184) -> ()  [unwired: 1 in, 2 out]
    }
  }
